vi "Configure Pressure Compensation.vi"(5 "Retry Attempts (0)":i32 min=0, 8 "error in":errorcluster, 10 "Pressure Compensation (PSI)":i32, 11 "VISA resource name":refnum<visa-resource-name>) -> (0 "error out":errorcluster, 3 "VISA resource name out":refnum<visa-resource-name>)   [LabVIEW 2020, in "ChromTech Series III Pump.lvlib"]
doc: "Stores the user flow rate compensation. Input range is 85.0 to 115.0 (i.e. +- 15.0 % compensation)."
uses:
  ChromTech Series III Pump.lvlib
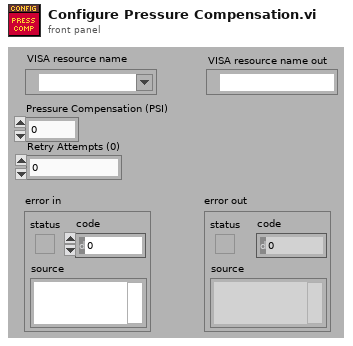
[diagram p1: front panel]
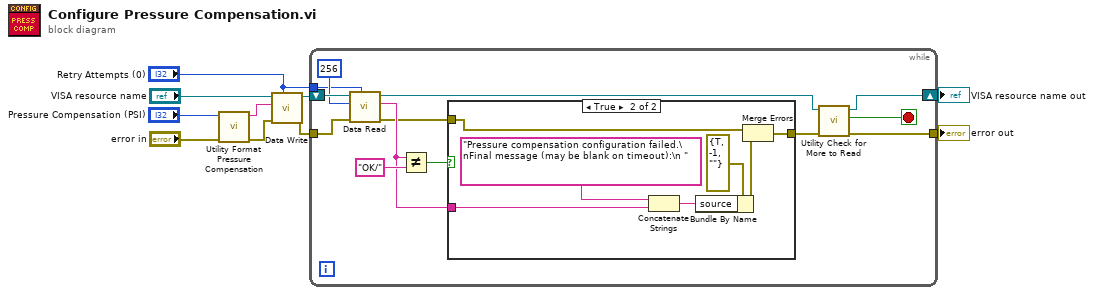
[diagram p0: block diagram]
diagram:
  n1 = call "Utility Format Pressure Compensation.vi"("error in (no error)"="error in", "Pressure Compensation (PSI)"="Pressure Compensation (PSI)") -> ("error out"=w5:errorcluster, "Formatted Compensation"=w4:string)  [unwired: 8 in]
  n2 = call "Data Write.vi"("Retry Attempts (0)"="Retry Attempts (0)", "error in (no error)"=w5, "Command"=w4, "VISA Refnum in"="VISA resource name") -> ("error out"=w8:errorcluster, "VISA Refnum out"=w9:refnum<visa-resource-name>)  [unwired: 6 in]
  n3 = while {
    tunnel: "Retry Attempts (0)" -> [w15]
    shift-right: [w12] -> w7
    shift-left: w9 -> [w23]
    tunnel: w8 -> [w22]
    tunnel: [w14] -> w2
    stop <- w11 stop-if-true
    n4 = call "Data Read.vi"("Retry Attempts (0)"=w15, "error in (no error)"=w22, "Bytes to read"=256, "VISA Refnum in"=w23) -> ("error out"=w17:errorcluster, "read buffer"=w18:string, "VISA Refnum out"=w13:refnum<visa-resource-name>)  [unwired: 5 in]
    n5 = Not Equal?(x=w18, y="OK/") -> (x != y?=w20:bool)
    n6 = case shown="True" w20 {
      tunnel: [w24 w30] -> w16
      tunnel: w17 -> [w24 w29]
      tunnel: w18 -> [_ w25]
      frame False {
      }
      frame True {
        n7 = Concatenate Strings("Pressure compensation configuration failed.\nFinal message (may be blank on timeout):\n ", w25) -> (w27:string)
        n8 = Bundle By Name(cluster=errorcluster {"status"=TRUE, "code"=-1, "source"=""} ("error out"), "source"=w27) -> (w28:errorcluster)
        n9 = Merge Errors(w29, w28) -> (w30:errorcluster)
      }
    }
    n10 = call "Utility Check for More to Read.vi"("error in (no error)"=w16, "VISA Refnum in"=w13) -> ("error out (unchanged)"=w14:errorcluster, "More to read?"=w11:bool, "VISA Refnum out"=w12:refnum<visa-resource-name>)  [unwired: 7 in]
  }
  "VISA resource name out" <- w7
  "error out" <- w2
